vi "OE1022D_Query_IDN.vi"(3 "错误输入（无错误）":errorcluster, 5 "VISA resource name":refnum<visa-resource-name>) -> (0 "错误输出":errorcluster, 1 "序列号":string, 2 "VISA resource name out":refnum<visa-resource-name>)   [LabVIEW 2022 SP3]
doc: "Configures the reference source and the internal oscillator."
panel:
  in  "数据转换":u8[](array[numeric])
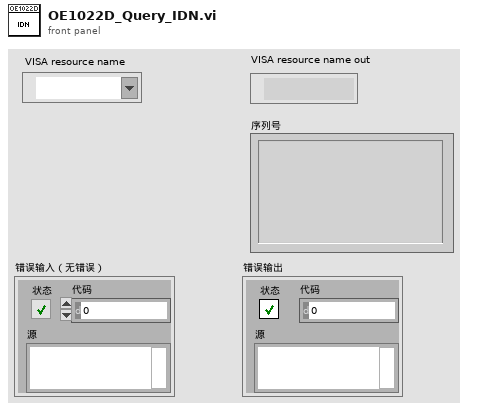
[diagram p1: front panel]
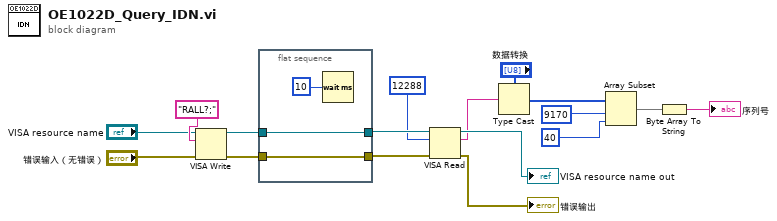
[diagram p0: block diagram]
diagram:
  n1 = VISA Write(VISA resource name="VISA resource name", write buffer="RALL?;" ("string (\"\")"), error in (no error)="错误输入（无错误）") -> (VISA resource name out=w17:refnum<visa-resource-name>, error out=w16:errorcluster)  [unwired: 1 out]
  n2 = flat-sequence {
    tunnel: [w19] -> w12
    tunnel: w17 -> [w19]
    tunnel: w16 -> [w18]
    tunnel: [w18] -> w11
    frame #0 {
      n3 = Wait (ms)(milliseconds to wait=u32 10 ("等待时间（毫秒）")) -> ()  [unwired: 1 out]
    }
  }
  n4 = VISA Read(VISA resource name=w12, byte count=12288, error in (no error)=w11) -> (VISA resource name out=→"VISA resource name out":refnum<visa-resource-name>, read buffer=w9:string, error out=→"错误输出":errorcluster)  [unwired: 1 out]
  n5 = Type Cast(type="数据转换", x=w9) -> (*(type *) &x=w7:u8[])
  n6 = Array Subset(array=w7, index=9170, length=40) -> (w4:u8[])
  n7 = Byte Array To String(unsigned byte array=w4) -> (string=→"序列号":string)
